vi "LINC Get LabVIEW Size.vi"(1 "bit size":i32, 2 "type":string) -> (0 "labview size":i32)   [LabVIEW 2018, in "STEPkgDriver_LINC.lvlib"]
uses:
  STEPkgDriver_LINC.lvlib
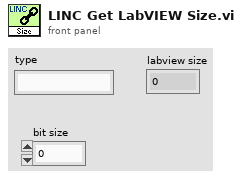
[diagram p1: front panel]
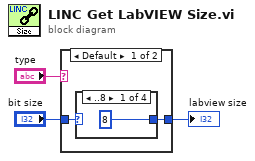
[diagram p0: block diagram]
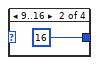
[diagram p2: hidden frame]
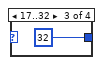
[diagram p3: hidden frame]
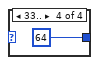
[diagram p4: hidden frame]
diagram:
  n1 = case shown="Default" "type" {
    tunnel: "bit size" -> [w5 w10]
    tunnel: [w4 w10] -> w1
    frame Default {
      n2 = case shown="..8" w5 {
        tunnel: [8 16 32 64] -> w4
        frame ..8 {
        }
        frame 9..16 {
        }
        frame 17..32 {
        }
        frame 33.. {
        }
      }
    }
    frame "STRING" {
    }
  }
  "labview size" <- w1
